vi "Teardown.vi"(11 "jettl Queue Actor in":refnum<class "jettl Queue Actor.lvclass">) -> (3 "jettl Queue Actor out":refnum<class "jettl Queue Actor.lvclass">)   [LabVIEW 2021, in "jettl.lvlib" / "jettl Queue Actor.lvclass"]
uses:
  jettl Queue Actor.lvclass
  C:/git/jettl/src/Queue Actor/Queue Actor.lvclass
  State/Teardown State/Teardown State.lvclass
  C:/git/jettl/src/jettl/State/State/State.lvclass
  jettl Queue Actor.lvclass/jettl Queue Actor.ctl
  State/State/State.lvclass
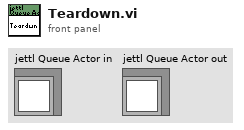
[diagram p1: front panel]
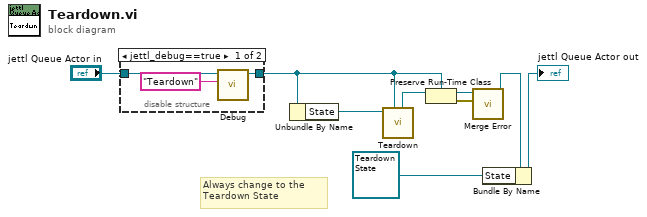
[diagram p0: block diagram]
diagram:
  # "Always change to the Teardown State"
  n1 = disable-structure shown="jettl_debug==true" {
    disable-tunnel: "jettl Queue Actor in" -> [w12 w13]
    disable-tunnel: [w11 w13] -> w1
    frame condition #0 (active) {
      n2 = call "Debug.vi"("Method"="Teardown", "jettl Queue Actor in"=w12) -> ("jettl Queue Actor out"=w11:refnum<class "jettl Queue Actor.lvclass">)  [unwired: 9 in]
    }
    frame condition #1 {
    }
  }
  n3 = Unbundle By Name(w1) -> ("State"=w8:refnum<class "State.lvclass">)
  n4 = call-dynamic "Teardown.vi"("Queue Actor in"=w1, "State in"=w8) -> ("Queue Actor out"=w6:refnum<class "Queue Actor.lvclass">)  [unwired: 9 in]
  n5 = Preserve Run-Time Class(object in=w6, 2:w1) -> (object out=w5:refnum<class "jettl Queue Actor.lvclass">, error out=w3:errorcluster)  [unwired: 1 in]
  n6 = call-dynamic "Merge Error.vi"("Error"=w3, "jettl Queue Actor in"=w5) -> ("jettl Queue Actor out"=w4:refnum<class "jettl Queue Actor.lvclass">)  [unwired: 9 in]
  n7 = Bundle By Name(cluster=w4, "State"=refnum<class "Teardown State.lvclass"> refnum ("LVCAM.lvlib:Destroying Self Actor State.lvclass")) -> (→"jettl Queue Actor out":refnum<class "jettl Queue Actor.lvclass">)
